vi "Web Browser.vi"() -> ()   [LabVIEW 2012]
uses:
  <vilib>/httpClient/LabVIEWHTTPClient.lvlib
panel:
  out "body":string
  in  "WebBrowser":refnum<k7>(container)
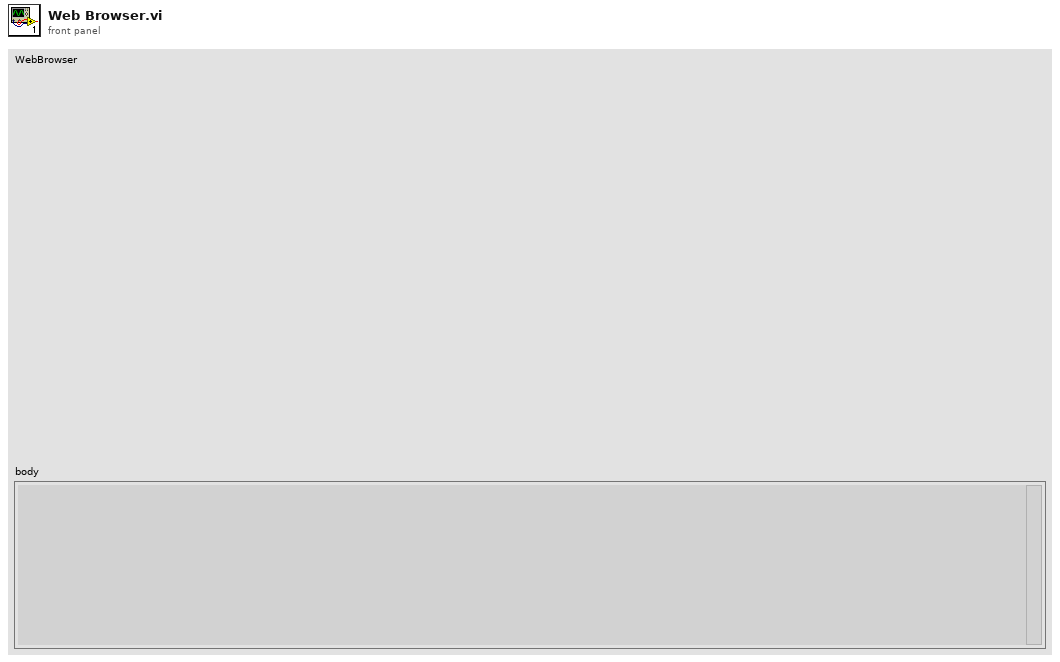
[diagram p1: front panel]
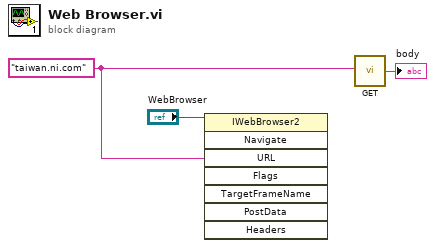
[diagram p0: block diagram]
diagram:
  w1 = "taiwan.ni.com" ("URL")
  n1 = invoke class="IWebBrowser2" method="Navigate"(reference="WebBrowser", "URL"=w1) -> ()  [unwired: 6 in, 8 out]
  n2 = call <vilib>:"GET.vi"("url"=w1) -> ("body"=→"body":string)  [unwired: 11 in, 3 out]
